vi "Change in Bundle Definition.vi"(8 "error in (no error)":errorcluster, 10 "Bundle Definition":T1, 11 "Bundle Builder in":refnum<class "Bundle Builder.lvclass">) -> (0 "error out":errorcluster, 1 "Custom Actions File Names":string[](array[string]), 2 "Product List File Names":string[](array[string]), 3 "Bundle Builder out":refnum<class "Bundle Builder.lvclass">, 4 "Bundle Filename":string)   [LabVIEW 2020, in "Bundle Builder.lvclass"]
uses:
  Bundle Builder.lvclass
  Bundle Builder.lvclass/Bundle Builder.ctl
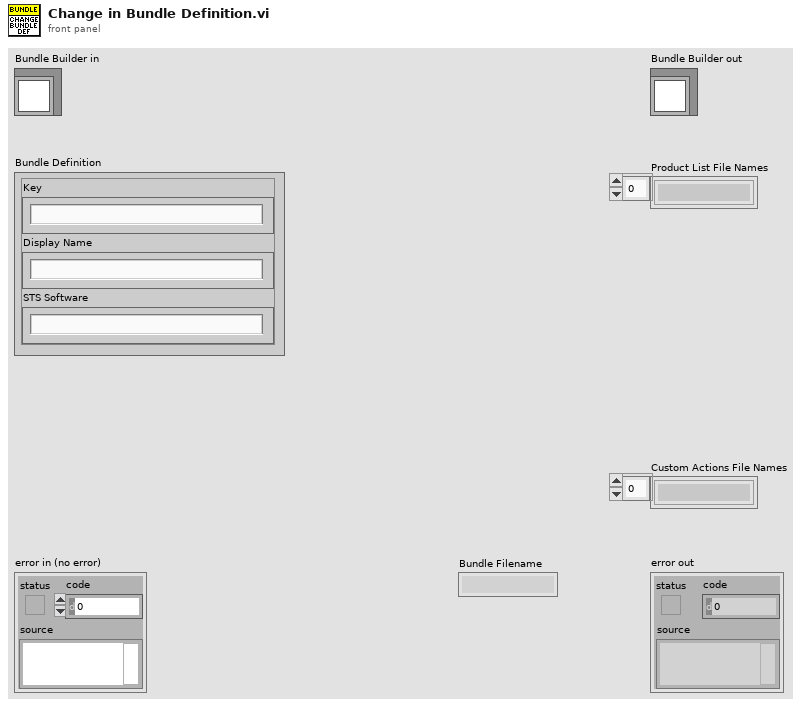
[diagram p1: front panel]
types:
  T1 = cluster{"Key":string, "Display Name":string, "STS Software":string}
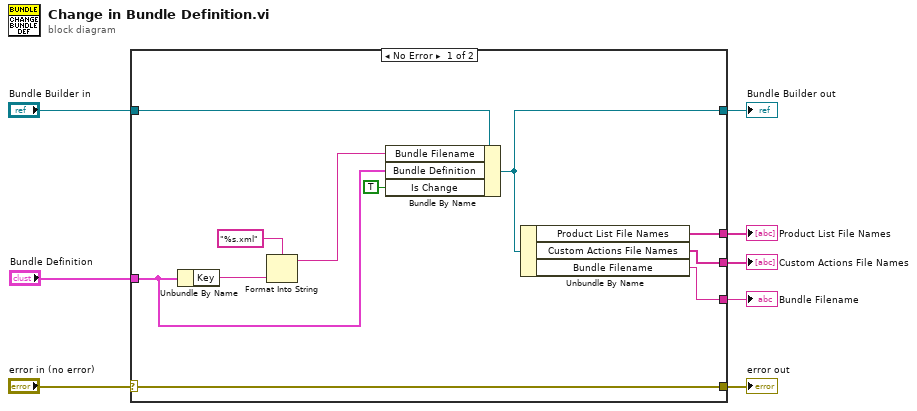
[diagram p0: block diagram]
diagram:
  n1 = case shown="No Error" "error in (no error)" {
    selector: "error in (no error)" -> [w19 w21]
    tunnel: [w19 w21] -> w7
    tunnel: [w17 w20] -> w5
    tunnel: "Bundle Builder in" -> [w18 w20]
    tunnel: "Bundle Definition" -> [w10 _]
    tunnel: [w16 _] -> w4
    tunnel: [w15 _] -> w3
    tunnel: [w14 _] -> w2
    frame No Error {
      n2 = Unbundle By Name(w10) -> ("Key"=w12:string)
      n3 = Format Into String(format string="%s.xml", w12) -> (resulting string=w11:string)  [unwired: 2 in, 1 out]
      n4 = Bundle By Name(cluster=w18, "Bundle Filename"=w11, "Bundle Definition"=w10, "Is Change"=TRUE) -> (w17:refnum<class "Bundle Builder.lvclass">)
      n5 = Unbundle By Name(w17) -> ("Product List File Names"=w16:string[], "Custom Actions File Names"=w15:string[], "Bundle Filename"=w14:string)
    }
    frame Error {
    }
  }
  "error out" <- w7
  "Bundle Builder out" <- w5
  "Product List File Names" <- w4
  "Custom Actions File Names" <- w3
  "Bundle Filename" <- w2
